vi "双控件移位.vi"(8 "错误输入（无错误）":errorcluster, 9 "终点控件":refnum<vi>, 10 "起始控件":refnum<vi>, 11 "需移动的控件":refnum<vi>) -> (0 "错误输出":errorcluster, 1 "终点控件输出":refnum<vi>, 2 "起始控件输出":refnum<vi>, 3 "移动控件输出":refnum<vi>)   [LabVIEW 8.6, in "窗口操作.lvlib"]
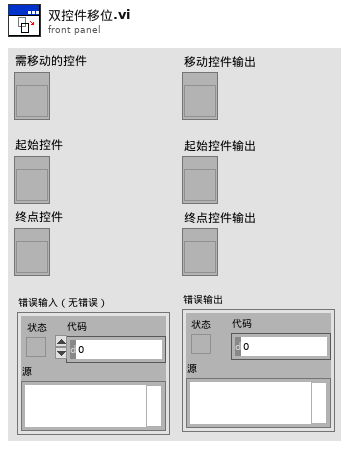
[diagram p1: front panel]
types:
  T1 = typedef "LVPositionTypeDef.ctl" = cluster{"Left":i32, "Top":i32}
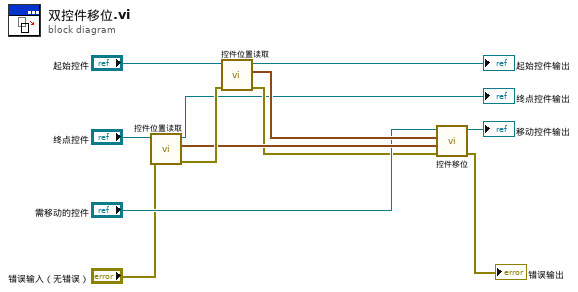
[diagram p0: block diagram]
diagram:
  n1 = call "控件位置读取.vi"("错误输入（无错误）"="错误输入（无错误）", "控件引用输入"="终点控件") -> ("错误输出"=w12:errorcluster, "位置"=w10:T1, "引用输出"=→"终点控件输出":refnum<vi>)  [unwired: 7 in]
  n2 = call "控件位置读取.vi"("错误输入（无错误）"=w12, "控件引用输入"="起始控件") -> ("错误输出"=w7:errorcluster, "位置"=w11:T1, "引用输出"=→"起始控件输出":refnum<vi>)  [unwired: 7 in]
  n3 = call "控件移位.vi"("错误输入（无错误）"=w7, "终点"=w10, "起始点"=w11, "控件引用输入"="需移动的控件") -> ("错误输出"=→"错误输出":errorcluster, "引用输出"=→"移动控件输出":refnum<vi>)  [unwired: 6 in]
